vi "Configure Channel.vi"(8 "error in (no error)":errorcluster, 10 "DAQmx Task In":refnum<k21>, 11 "IEPEChannel in":refnum<class "IEPEChannel.lvclass">) -> (0 "error out":errorcluster, 2 "DAQmx Task":refnum<k21>)   [LabVIEW 2020, in "VolatusDAQConfig.lvlib" / "IEPEChannel.lvclass"]
uses:
  IEPEChannel.lvclass
  IEPEChannel.lvclass/IEPEChannel.ctl
  VolatusConfig/VolatusConfigElement/VolatusConfigElement.lvclass
  VolatusConfig/Channel/Channel.lvclass
  C:/dev/lv20CE/relink/lv-volatus/VolatusDAQConfig/DAQmxChannel/DAQmxChannel.lvclass
  C:/dev/lv20CE/relink/lv-volatus/VolatusConfig/Channel/Channel.lvclass
  C:/dev/lv20CE/relink/lv-volatus/VolatusConfig/VolatusConfigElement/VolatusConfigElement.lvclass
  C:/dev/lv20CE/relink/lv-volatus/VolatusDAQConfig/IEPEChannel/IEPEChannel.lvclass
  <vilib>/DAQmx/create/channels.llb/DAQmx Create Channel (AI-Acceleration-Accelerometer).vi
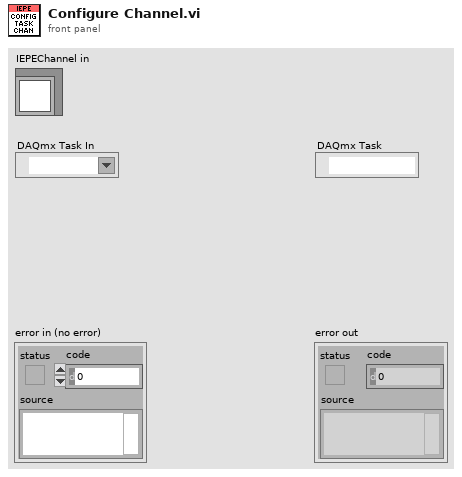
[diagram p1: front panel]
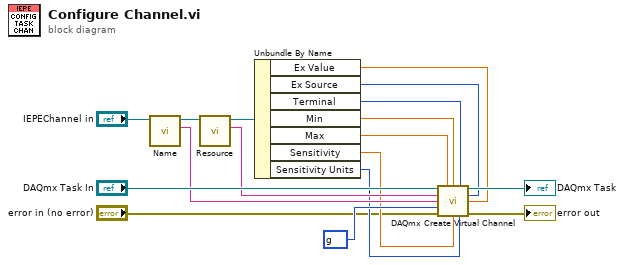
[diagram p0: block diagram]
diagram:
  w11 = 10186 items=["g"=10186, "m/s^2"=12470, "in/s^2"=12471, "From Custom Scale"=10065] ("units")
  n1 = call "Name.vi"("VolatusConfigElement in"="IEPEChannel in") -> ("Name"=w12:string, "VolatusConfigElement out"=w15:refnum<class "IEPEChannel.lvclass">)  [unwired: 8 in, 1 out]
  n2 = call "Resource.vi"("Channel in"=w15) -> ("Resource"=w13:string, "Channel out"=w10:refnum<class "IEPEChannel.lvclass">)  [unwired: 8 in, 1 out]
  n3 = Unbundle By Name(w10) -> ("Ex Value"=w5:dbl, "Ex Source"=w6:i32, "Terminal"=w9:i32, "Min"=w8:dbl, "Max"=w7:dbl, "Sensitivity"=w4:dbl, "Sensitivity Units"=w3:i32)
  n4 = call-poly <vilib>:"DAQmx Create Virtual Channel.vi"("task in"="DAQmx Task In", "maximum value"=w7, "minimum value"=w8, "input terminal configuration"=w9, "physical channels"=w13, "current excitation source"=w6, "name to assign"=w12, "current excitation value"=w5, "units"=w11, "error in"="error in (no error)", "sensitivity"=w4, "sensitivity units"=w3) -> ("task out"=→"DAQmx Task":refnum<k21>, "error out"=→"error out":errorcluster)  [unwired: 2 in]
